vi "QImaging_Main.vi"() -> ()   [LabVIEW 2014]
uses:
  QImaging_Basic/Controls/Readout Speed.ctl
  QImaging_Basic/Controls/Parameter.ctl
  Release/QImaging.dll
panel:
  out "ConfigCam err Readout":i32
  out "ConfigCam err Hi Sens":i32
  in  "High Sensitivity":bool=TRUE
  in  "Readout Speed":T1
  out "Message":string
  in  "Stop Live Preview":bool
  in  "Abort Multi Grab":bool
  in  "Multi Grab":bool
  out "Saturating?":bool
  out "Average":dbl
  out "Std Dev":dbl
  in  "Overwrite?":bool
  in  "Snap current Data":bool
  in  "Save Data":bool
  in  "Racine chemin de sauvegarde":path=path "C:/Users/loa/Documents/DONNEES MANIP GAZ/Hiver 2015"
  out "Warning":bool
  out "Message":string
  in  "Indice":u32
  in  "Nom du fichier":string="tir"
  in  "Mode de Sauvegarde":u16(ring)=1 items=["Manuel", "Automatique"]
  out "Max Val":u16
  out "CCD Height":u32=1 min=1 max=4 step=1
  out "CCD Width":u32=1 min=1 max=4 step=1
  out "Camera Handle":u32
  in  "Abort Frame":bool
  out "sizeOfBuf":u32
  out "errcode":i32
  out "pBuf address":u32
  out "pFrame address":u32
  out "Waiting for Trigger":bool
  in  "Grab Image":bool
  in  "Queue Frame":bool
  in  "Trig":bool
  out "ROI Height":u32=1 min=1 max=4 step=1
  out "ROI Width":u32=1 min=1 max=4 step=1
  in  "Binning":u32=1 min=1 max=4 step=1
  out "ParamVal":u32[](array[numeric])
  out "Open Cam Error":i32
  out "LibCam Error":u32
  out "LibOpen error":i32
  in  "Exposure Time":u32=100
  out "Camera Id":u32
  out "error out":errorcluster
  in  "error in (no error)":errorcluster
  in  "Stop":bool
  out "Captured Image":u16[][](graph)
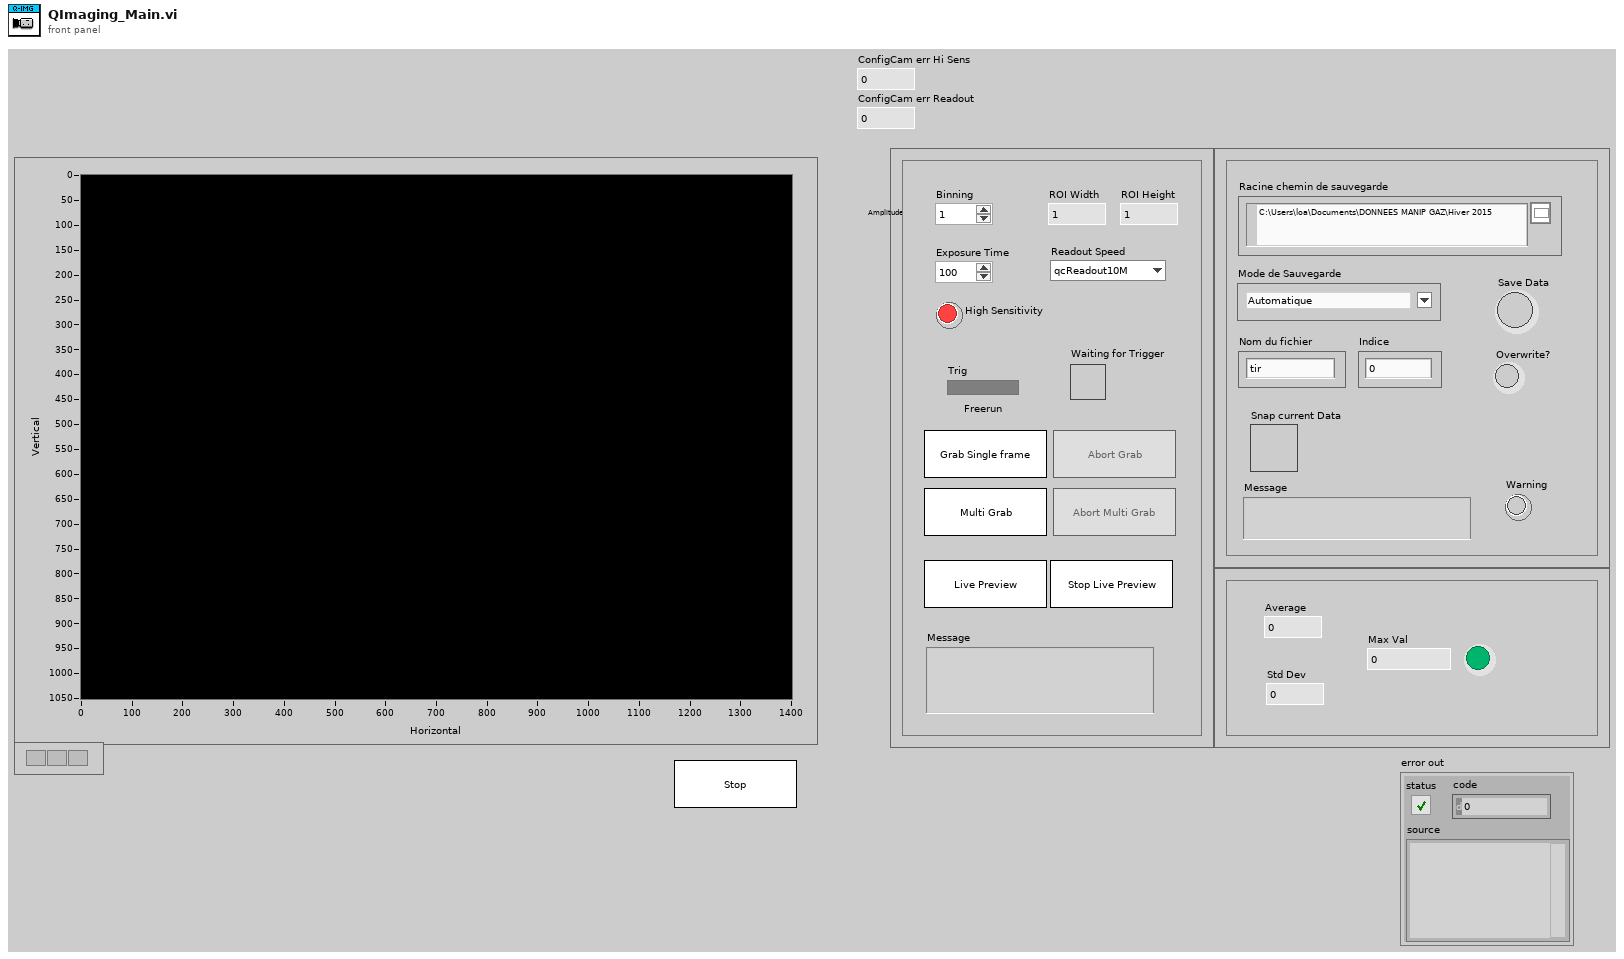
[diagram p1: front panel]
types:
  T1 = typedef "Readout Speed.ctl" = enum16{"qcReadout10M", "qcReadout20M", "qcReadout30M"}
  T2 = enum8{"Enabled", "Disabled", "Disabled and Grayed Out"}
  T3 = typedef "Parameter.ctl" = enum32{"Gain ", "Offset", "Exposure", "Binning", "HzBinning", "VtBinning", "Readout speed", "Trigger Type", "Color Wheel", "Cooler Active", "Exposure red", "Exposure blue", "Image format", "ROI X", "ROI Y", "ROI Width", "ROI Height", "Reserved1", "Shutter State", "Reserved2", "SyncB", "Reserved3", "IntensifierGain (deprecated)", "Trig Delay", "Camera Mode", "Normalized Gain", "Normalized Intensifier Gain", "Do post processing ", "Post Proc Gain Red", "Post Proc Gain Green", "Post Proc Gain Blue", "Post Proc Bayer Algo", "Post Proc Image Format", "Fan Speed", "Blackout Mode", "High Sensitivity Mode", "Readout Port", "EM Gain", "Open Delay Shutter", "Close Delay Shutter", "CCD Clearing Mode", "Over Sample", "Reserved5", "Reserved6", "Reserved7"}
  T4 = typedef "Image Type" = u32
  T5 = typedef "IMAQ Image.ctl" = refnum<image>
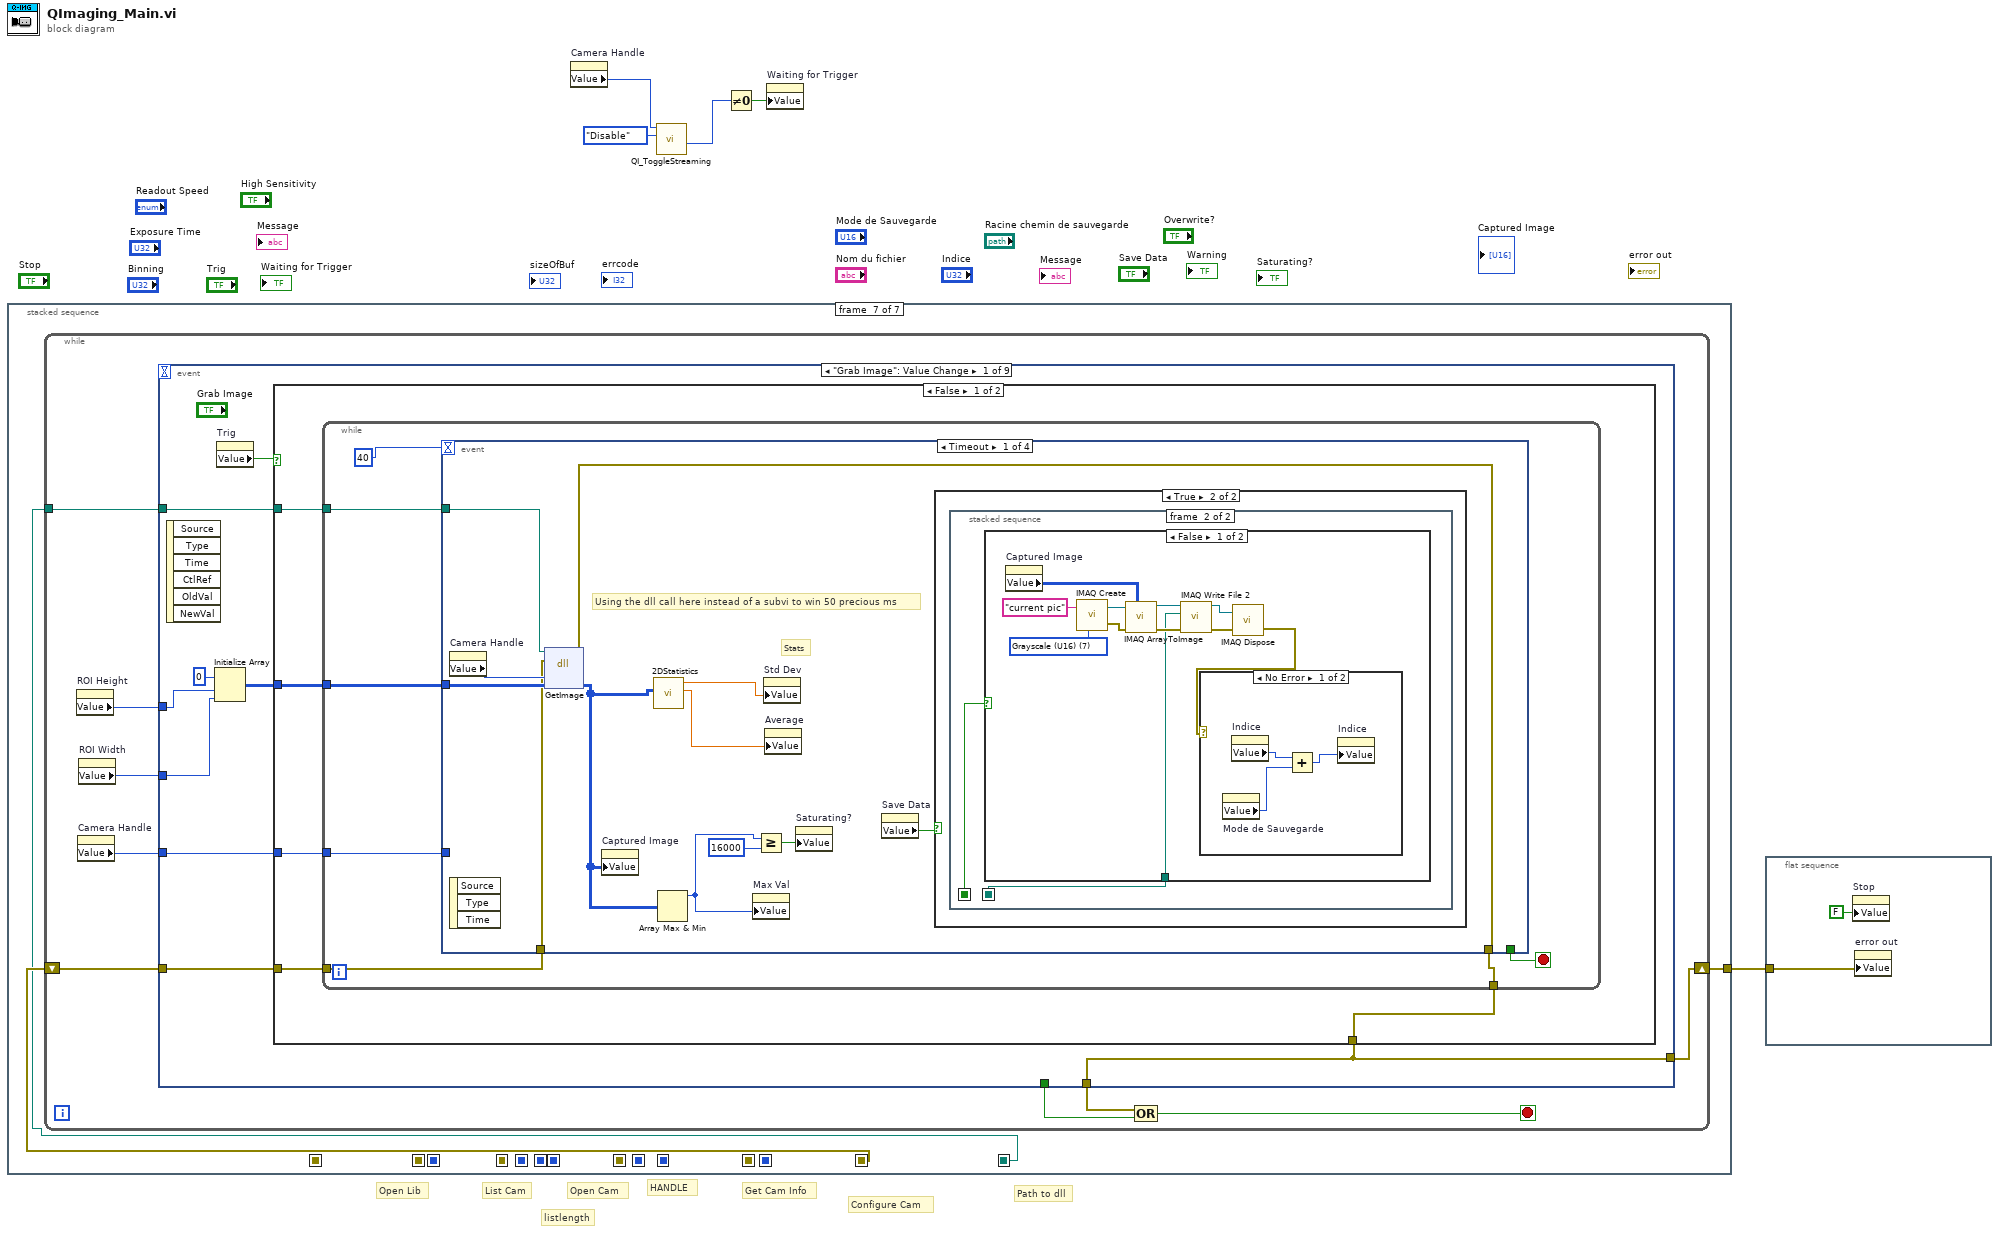
[diagram p0: block diagram]
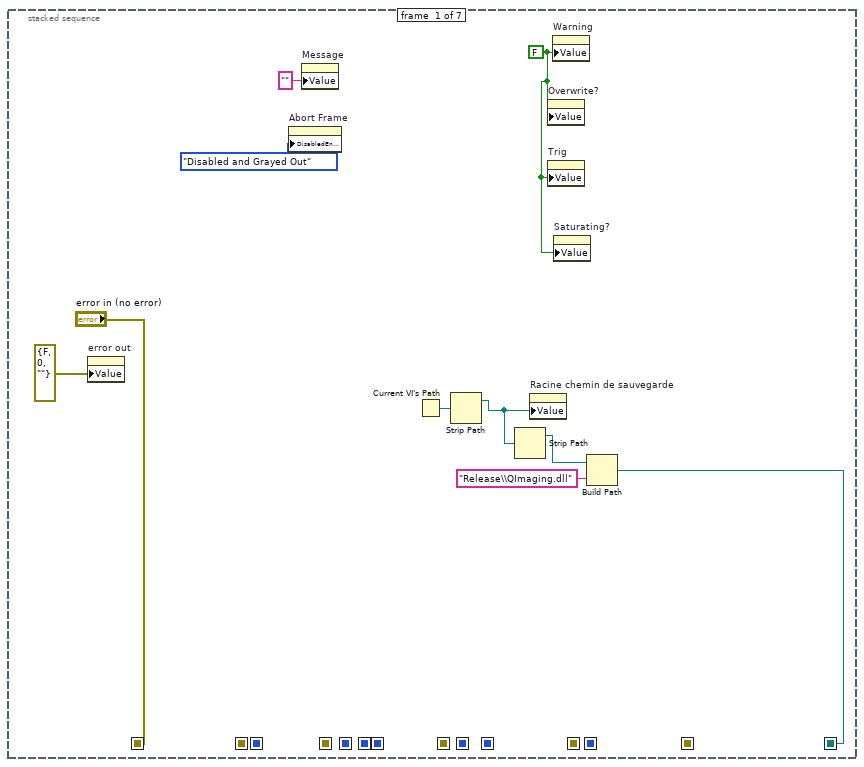
[diagram p2: hidden frame]
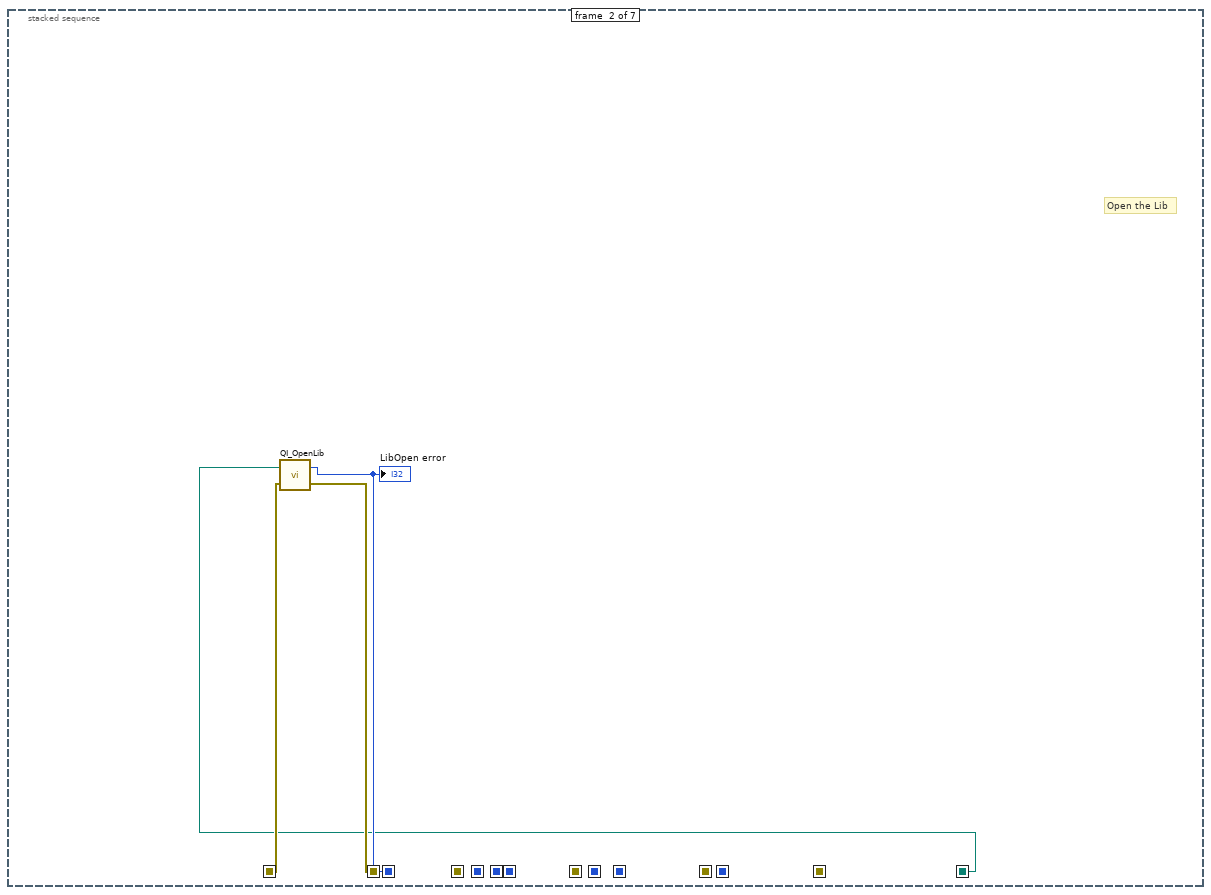
[diagram p3: hidden frame]
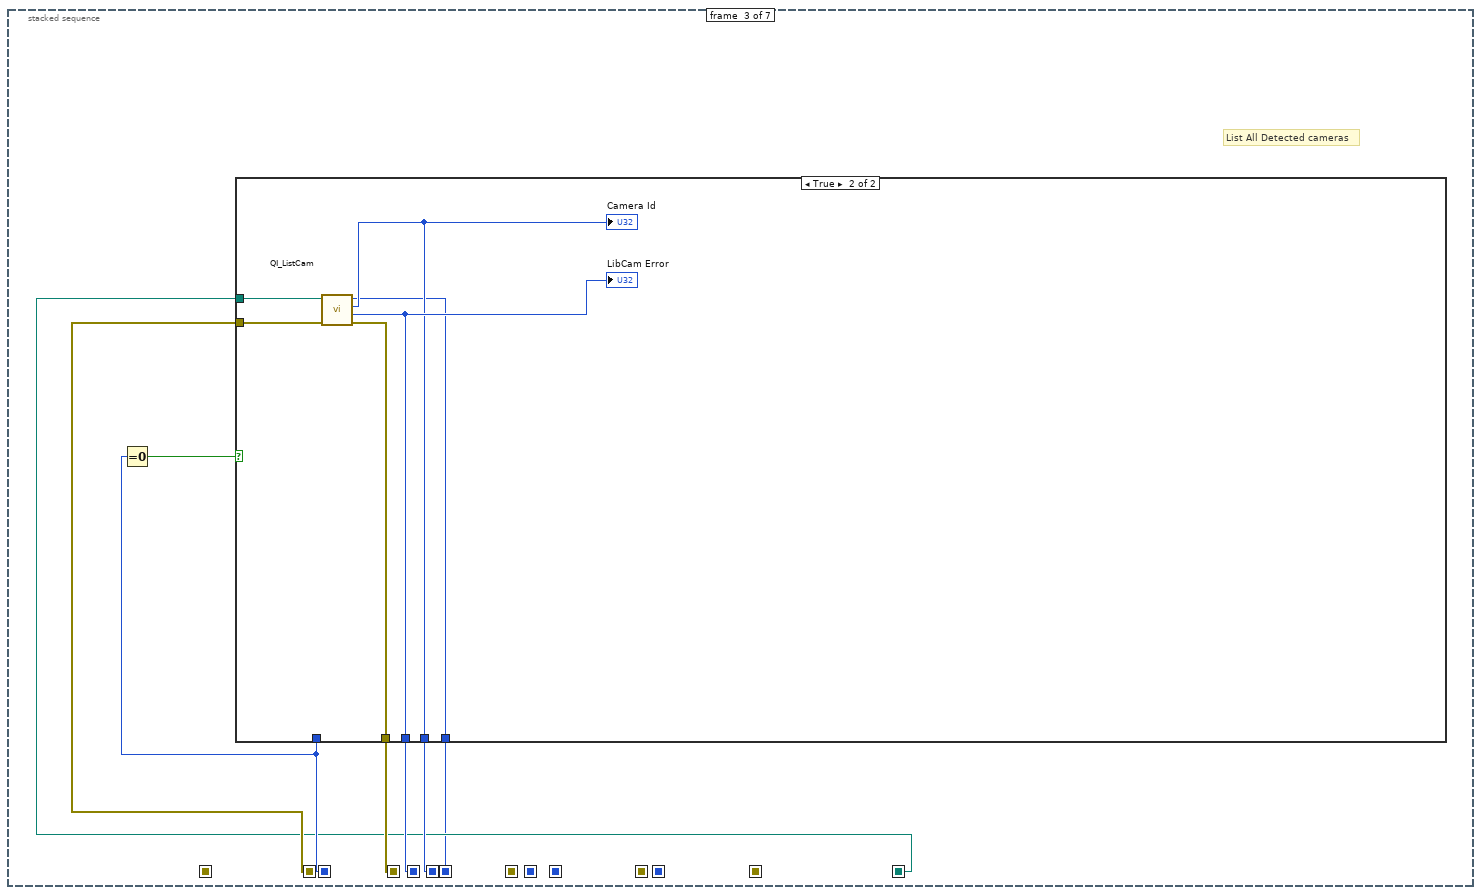
[diagram p4: hidden frame]
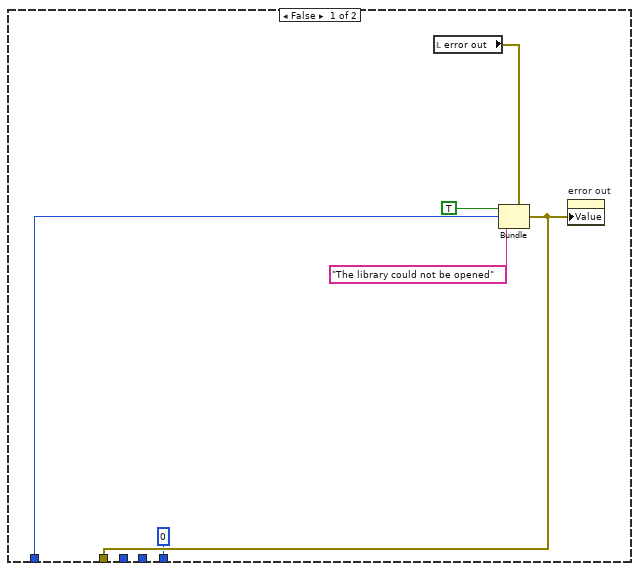
[diagram p5: hidden frame]
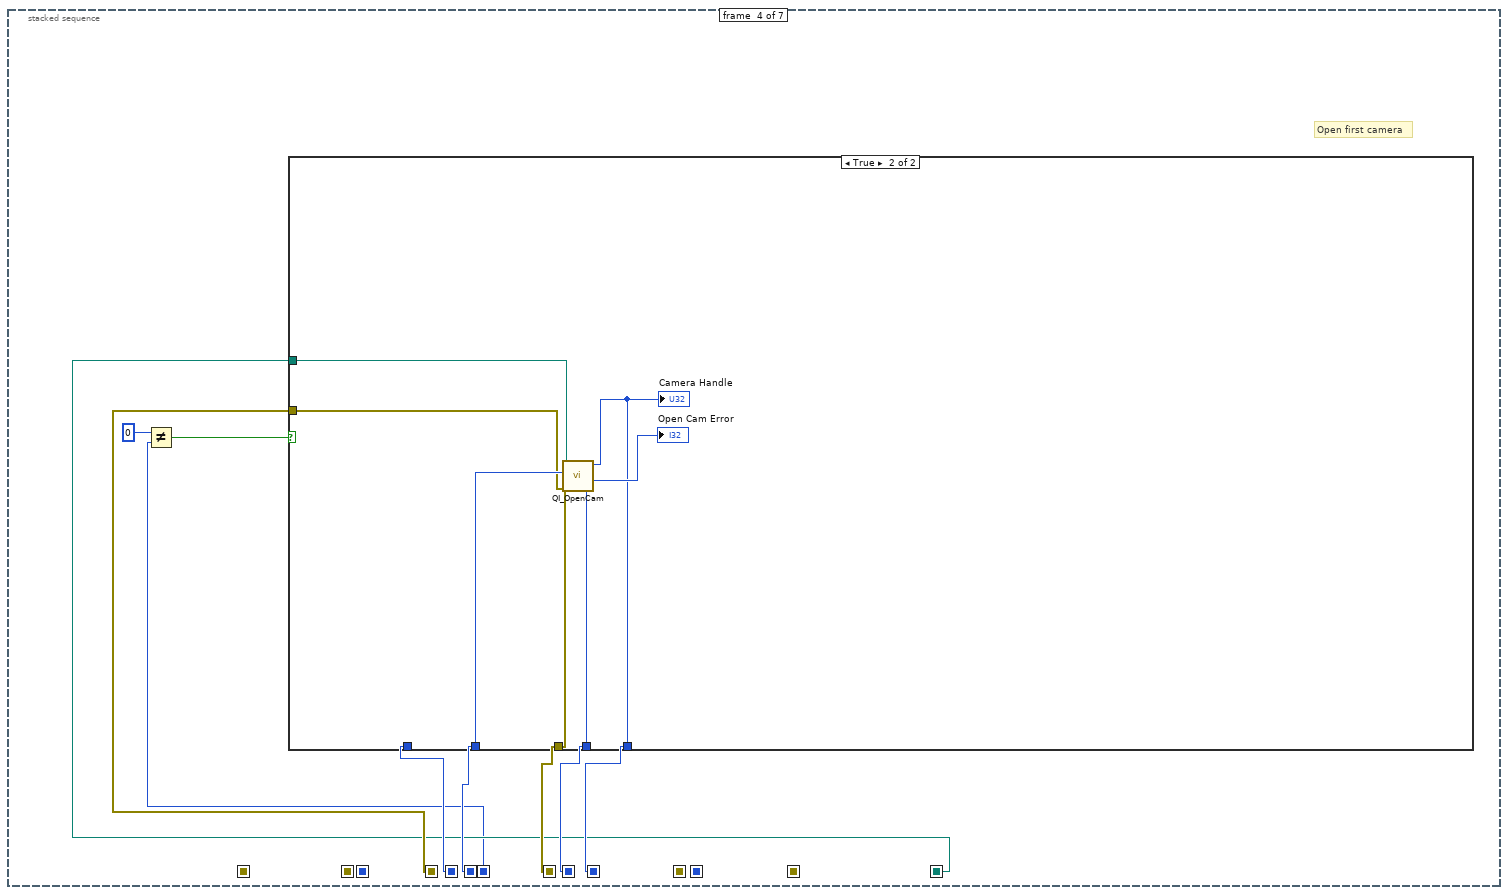
[diagram p6: hidden frame]
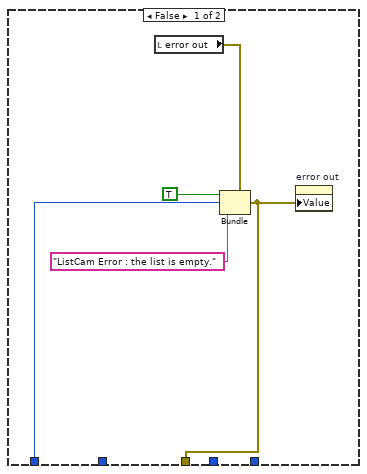
[diagram p7: hidden frame]
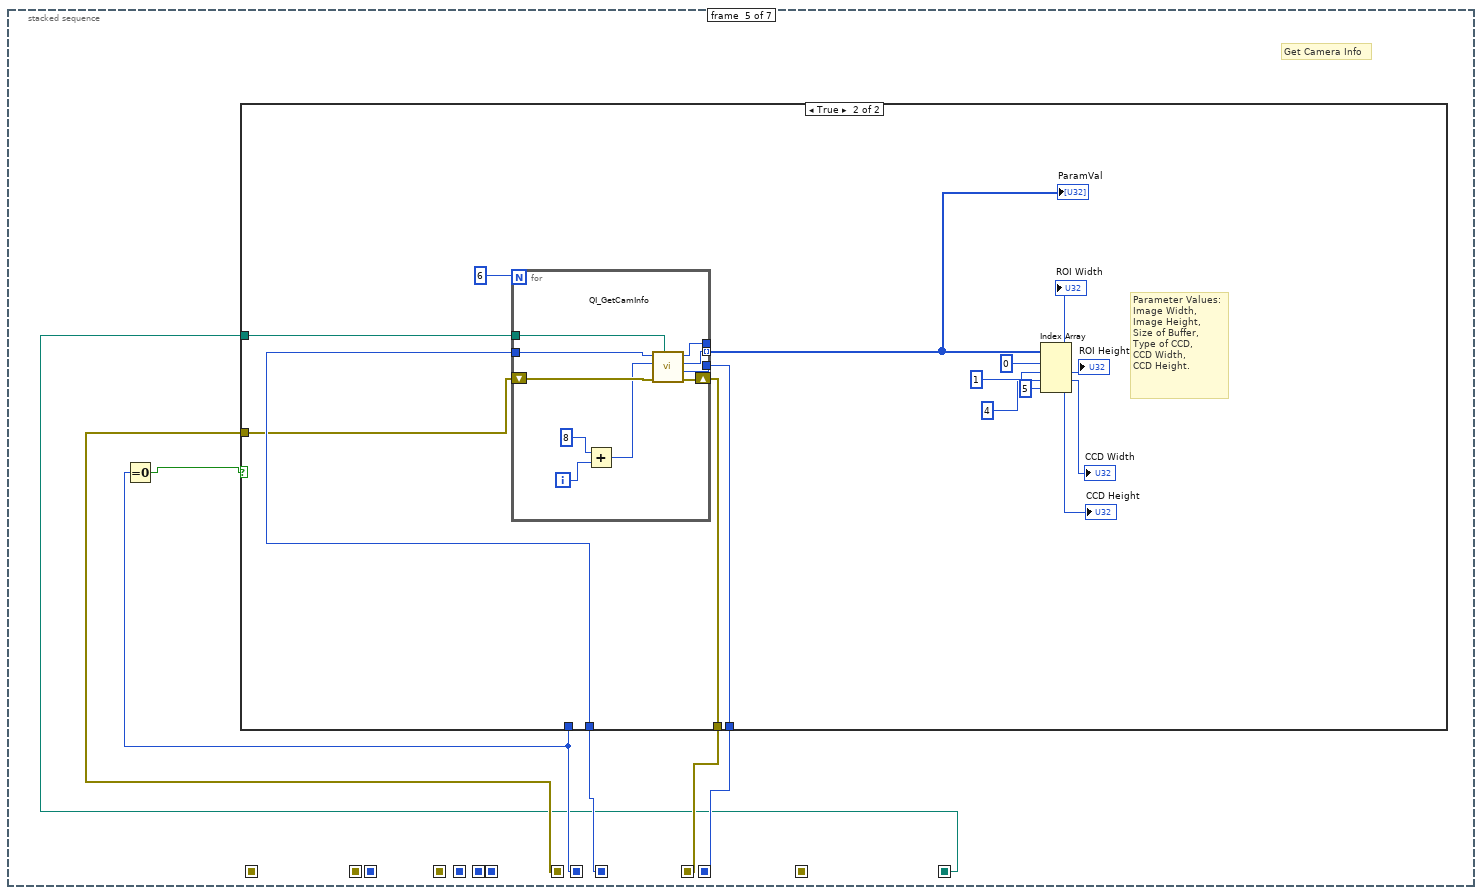
[diagram p8: hidden frame]
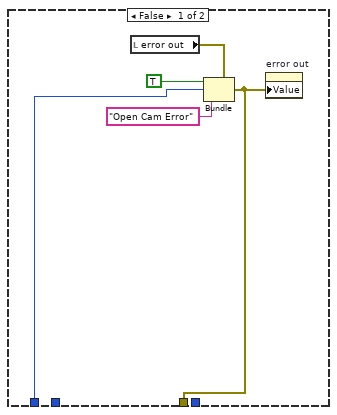
[diagram p9: hidden frame]
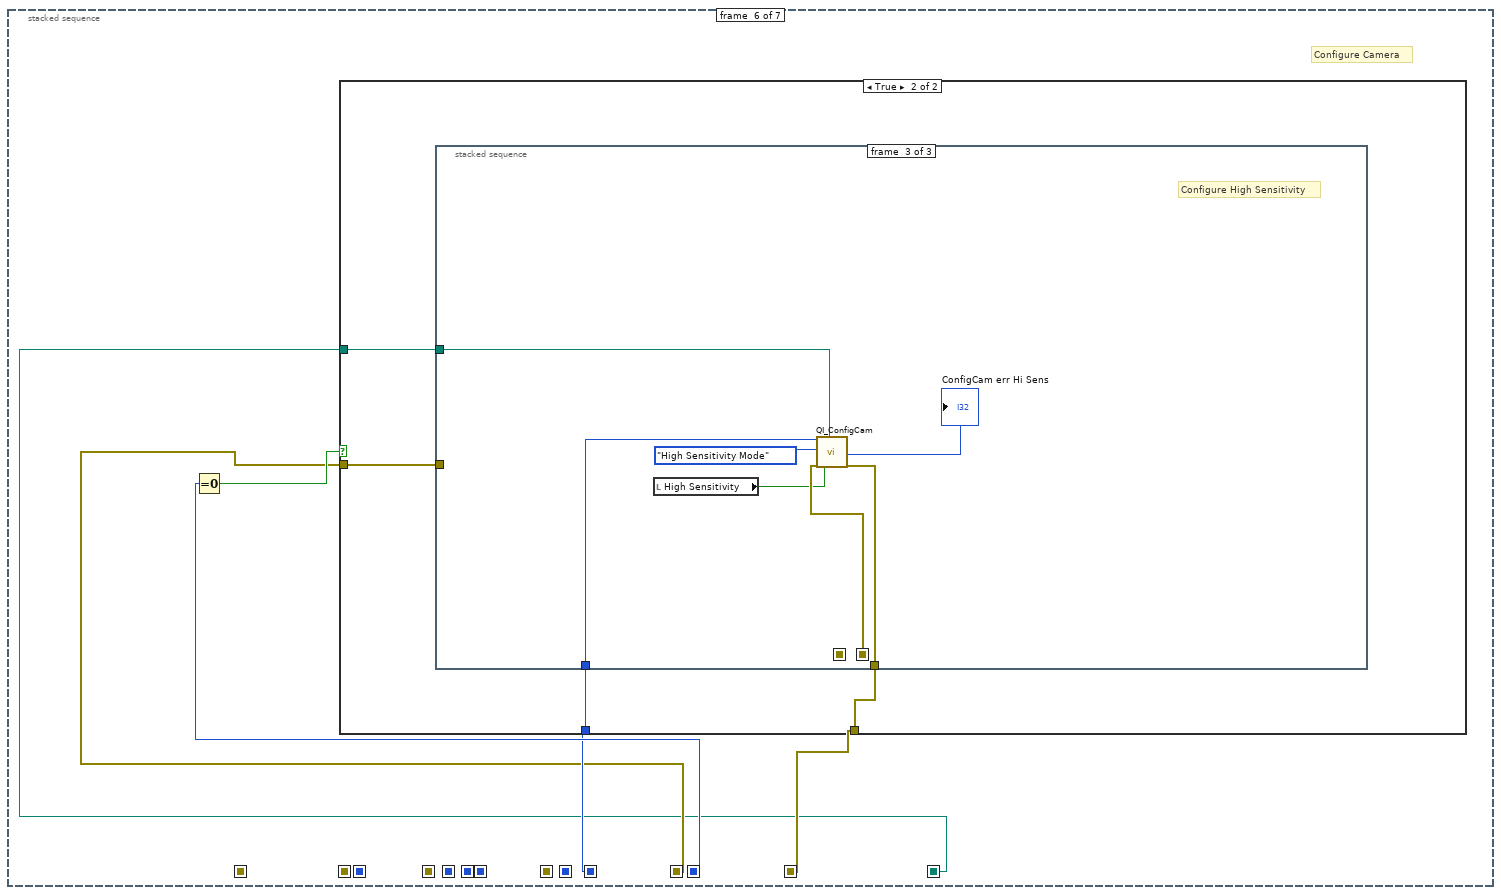
[diagram p10: hidden frame]
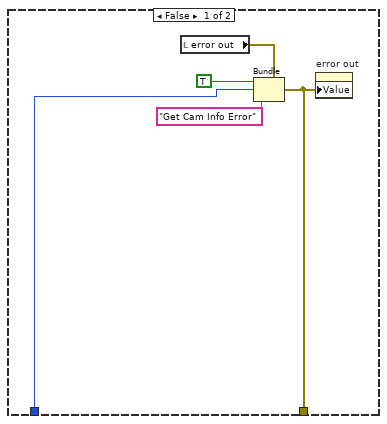
[diagram p11: hidden frame]
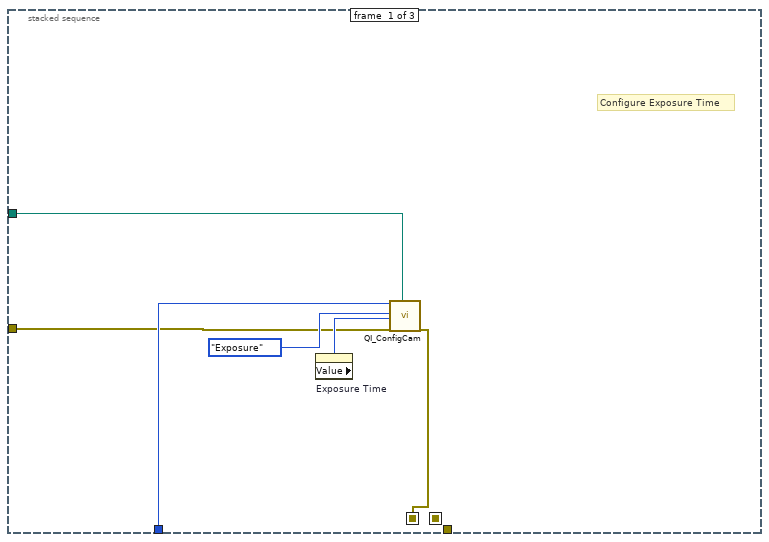
[diagram p12: hidden frame]
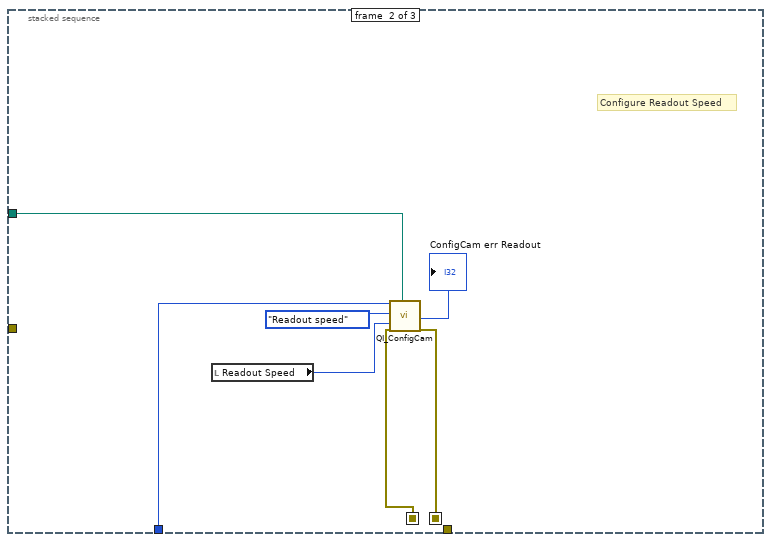
[diagram p13: hidden frame]
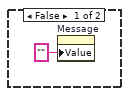
[diagram p14: hidden frame]
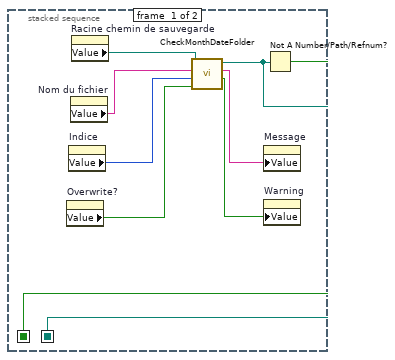
[diagram p15: hidden frame]
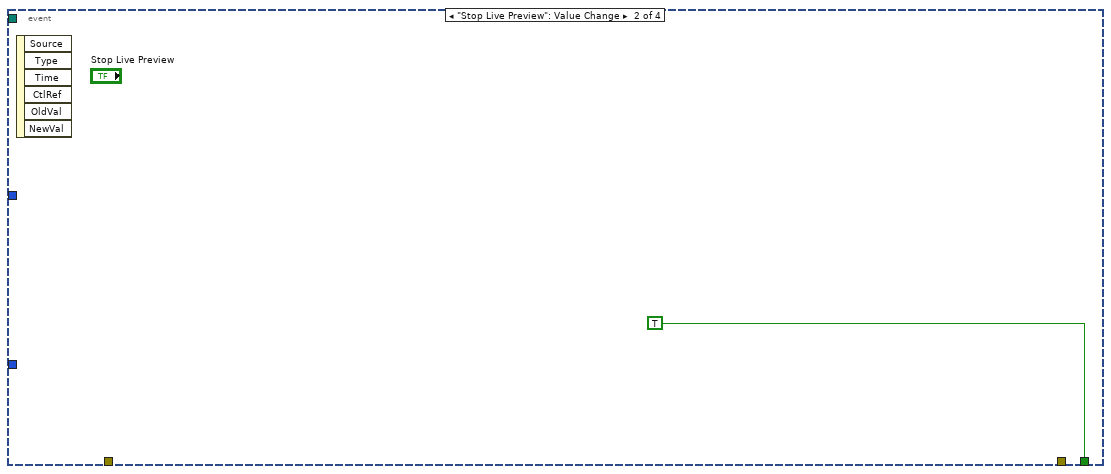
[diagram p18: hidden frame]
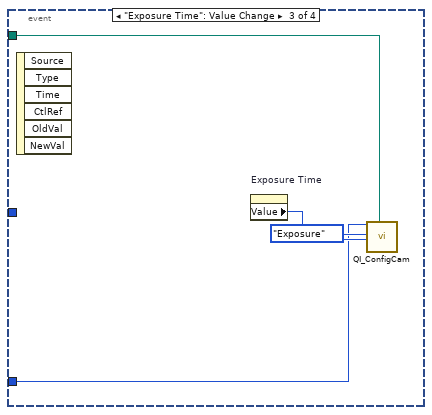
[diagram p19: hidden frame]
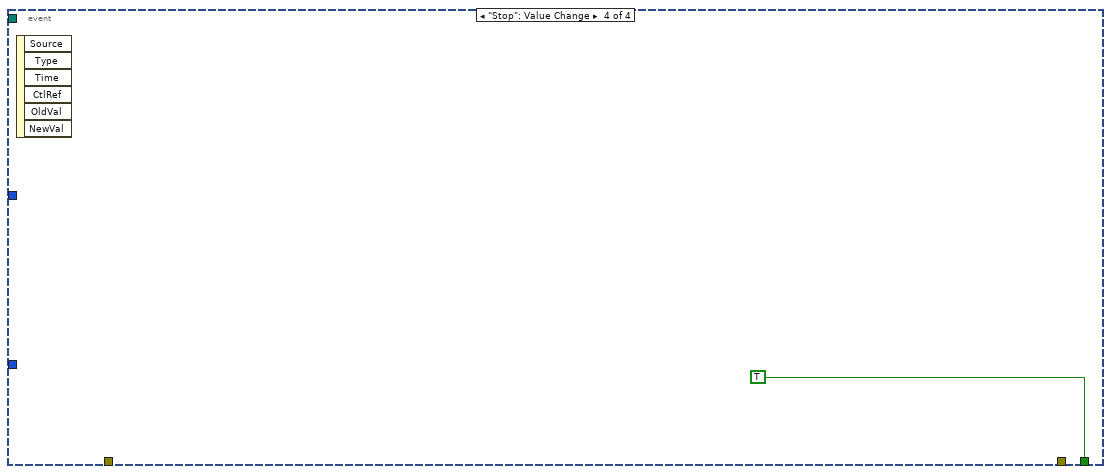
[diagram p20: hidden frame]
diagram:
  # "listlength"
  # "Path to dll"
  # "HANDLE"
  # "Configure Cam"
  # "Get Cam Info"
  # "Open Cam"
  # "List Cam"
  # "Open Lib"
  n1 = stacked-sequence {
    seq-local: [_ w19 _ _ _ _ _] -> [_ _ w22 _ _ _ _]
    seq-local: [_ w18 _ _ _ _ _] -> [_ _ w24 _ _ _ _]
    seq-local: [_ _ w27 _ _ _ _] -> [_ _ _ w43 _ _ _]
    seq-local: [_ _ w26 _ _ _ _] -> [_ _ _ w45 _ _ _]
    seq-local: [_ _ w25 _ _ _ _] -> [_ _ _ w49 _ _ _]
    seq-local: [_ _ _ w48 _ _ _] -> [_ _ _ _ w62 _ _]
    seq-local: [_ _ _ w47 _ _ _] -> [_ _ _ _ w64 _ _]
    seq-local: [_ _ _ w46 _ _ _] -> [_ _ _ _ w67 w102 _]
    seq-local: [_ _ _ _ w66 _ _] -> [_ _ _ _ _ w99 _]
    seq-local: [_ _ _ _ w65 _ _] -> [_ _ _ _ _ w103 _]
    seq-local: [_ _ _ _ _ w101 _] -> [_ _ _ _ _ _ w135]
    seq-local: ["error in (no error)" _ _ _ _ _ _] -> [_ w17 _ _ _ _ _]
    seq-local: [w6 _ _ _ _ _ _] -> [_ w16 w21 w42 w61 w98 w133]
    seq-local: [_ _ w20 _ _ _ _] -> [_ _ _ w41 _ _ _]
    tunnel: [_ _ _ _ _ _ w134] -> w5
    frame #0 {
      w11 = FALSE ("Warning")
      n2 = property on="error out" class="Clust (strict)"("Value"=errorcluster {"status"=FALSE, "code"=0, "source"=""} ("error in (no error)")) -> ()  [unwired: 2 in, 2 out]
      n3 = property on="Abort Frame" class="Bool"("DisabledEnum"=T2."Disabled and Grayed Out" ("Disabled")) -> ()  [unwired: 2 in, 2 out]
      n4 = property on="Message" class="Str"("Value"="" ("Message")) -> ()  [unwired: 2 in, 2 out]
      n5 = Current VI's Path() -> (path=w10:path)
      n6 = Strip Path(path=w10) -> (stripped path=w9:path)  [unwired: 1 out]
      n7 = Strip Path(path=w9) -> (stripped path=w8:path)  [unwired: 1 out]
      n8 = property on="Racine chemin de sauvegarde" class="Path"("Value"=w9) -> ()  [unwired: 2 in, 2 out]
      n9 = property on="Overwrite?" class="Bool (strict)"("Value"=w11) -> ()  [unwired: 2 in, 2 out]
      n10 = property on="Trig" class="Bool (strict)"("Value"=w11) -> ()  [unwired: 2 in, 2 out]
      n11 = property on="Warning" class="Bool (strict)"("Value"=w11) -> ()  [unwired: 2 in, 2 out]
      n12 = property on="Saturating?" class="Bool (strict)"("Value"=w11) -> ()  [unwired: 2 in, 2 out]
      n13 = Build Path(base path=w8, name or relative path="Release\\QImaging.dll") -> (appended path=w6:path)
    }
    frame #1 {
      # "Open the Lib"
      n14 = call "QI_OpenLib.vi"("error in (no error)"=w17, "path to dll"=w16) -> ("error out"=w19:errorcluster, "LibOpen error"=w18:i32)
      "LibOpen error" <- w18
    }
    frame #2 {
      # "List All Detected cameras"
      n15 = Equal To 0?(x=w24) -> (x = 0?=w23:bool)
      n16 = case shown="True" w23 {
        tunnel: w24 -> [w30 _]
        tunnel: [w29 w39] -> w27
        tunnel: [_ w38] -> w26
        tunnel: [_ w37] -> w25
        tunnel: w22 -> [_ w36]
        tunnel: w21 -> [_ w35]
        tunnel: [u32 0 ("listLength") w34] -> w20
        frame False {
          n17 = local read "error out"() -> (w31:errorcluster)
          n18 = Bundle(cluster=w31, "status"=TRUE, "code"=w30, "source"="The library could not be opened") -> (w29:errorcluster)
          n19 = property on="error out" class="Clust (strict)"("Value"=w29) -> ()  [unwired: 2 in, 2 out]
        }
        frame True {
          n20 = call "QI_ListCam.vi"("error in (no error)"=w36, "path to dll"=w35) -> ("error out"=w39:errorcluster, "LibCam Error"=w38:u32, "cameraId"=w37:u32, "listLength"=w34:u32)  [unwired: 6 in]
          "Camera Id" <- w37
          "LibCam Error" <- w38
        }
      }
    }
    frame #3 {
      # "Open first camera"
      n21 = Not Equal?(x=u32 0, y=w41) -> (x != y?=w44:bool)
      n22 = case shown="True" w44 {
        tunnel: w49 -> [_ w60]
        tunnel: [w50 w59] -> w48
        tunnel: [_ w58] -> w47
        tunnel: [_ w57] -> w46
        tunnel: w45 -> [w51 _]
        tunnel: w43 -> [_ w56]
        tunnel: w42 -> [_ w55]
        frame False {
          n23 = local read "error out"() -> (w52:errorcluster)
          n24 = Bundle(cluster=w52, "status"=TRUE, "code"=w51, "source"="ListCam Error : the list is empty.") -> (w50:errorcluster)
          n25 = property on="error out" class="Clust (strict)"("Value"=w50) -> ()  [unwired: 2 in, 2 out]
        }
        frame True {
          n26 = call "QI_OpenCam.vi"("error in (no error)"=w56, "Camera ID"=w60, "path to dll"=w55) -> ("error out"=w59:errorcluster, "Open Cam Error"=w58:i32, "Camera Handle"=w57:u32)  [unwired: 6 in]
          "Camera Handle" <- w57
          "Open Cam Error" <- w58
        }
      }
    }
    frame #4 {
      # "Get Camera Info"
      n27 = Equal To 0?(x=w64) -> (x = 0?=w63:bool)
      n28 = case shown="True" w63 {
        tunnel: w67 -> [_ w82]
        tunnel: [w68 w81] -> w66
        tunnel: w64 -> [w69 _]
        tunnel: [_ w80] -> w65
        tunnel: w62 -> [_ w79]
        tunnel: w61 -> [_ w73]
        frame False {
          n29 = local read "error out"() -> (w70:errorcluster)
          n30 = Bundle(cluster=w70, "status"=TRUE, "code"=w69, "source"="Open Cam Error") -> (w68:errorcluster)
          n31 = property on="error out" class="Clust (strict)"("Value"=w68) -> ()  [unwired: 2 in, 2 out]
        }
        frame True {
          # "Parameter Values:\nImage Width,\nImage Height,\nSize of Buffer,\nType of CCD,\nCCD Width,\nCCD Height."
          n32 = for {
            N: 6 -> [_]
            shift-right: [w93] -> w81
            shift-left: w79 -> [w97]
            tunnel: [w92] -> _
            tunnel: [w91] -> w84 mode=indexing
            tunnel: [w90] -> w80
            tunnel: w82 -> [w89]
            tunnel: w73 -> [w88]
            i -> [w96]
            n33 = Add(x=u32 8, y=w96) -> (x+y=w94:u32)
            n34 = call "QI_GetCamInfo.vi"("path to dll"=w88, "error in (no error)"=w97, "paramKey"=w94, "Camera Handle"=w89) -> ("error out"=w93:errorcluster, "CamInfo err"=w90:i32, "paramVal"=w91:u32, "Camera Handle"=w92:u32)  [unwired: 4 in]
          }
          "ParamVal" <- w84
          n35 = Index Array(array=w84, index #1=0 ("index"), index #2=1 ("index"), index #3=4 ("index"), index #4=5 ("index")) -> (element #1=→"ROI Width":u32, element #2=→"ROI Height":u32, element #3=→"CCD Width":u32, element #4=→"CCD Height":u32)
        }
      }
    }
    frame #5 {
      # "Configure Camera"
      n36 = Equal To 0?(x=w103) -> (x = 0?=w100:bool)
      n37 = case shown="True" w100 {
        tunnel: w102 -> [w105 w112]
        tunnel: [w104 w109] -> w101
        tunnel: w99 -> [_ w111]
        tunnel: w98 -> [_ w110]
        frame False {
          n38 = local read "error out"() -> (w106:errorcluster)
          n39 = Bundle(cluster=w106, "status"=TRUE, "code"=w105, "source"="Get Cam Info Error") -> (w104:errorcluster)
          n40 = property on="error out" class="Clust (strict)"("Value"=w104) -> ()  [unwired: 2 in, 2 out]
        }
        frame True {
          n41 = stacked-sequence {
            seq-local: [w113 _ _] -> [_ w122 _]
            seq-local: [_ w121 _] -> [_ _ w129]
            tunnel: w112 -> [w116 w124 w131]
            tunnel: w111 -> [w115 _ _]
            tunnel: w110 -> [w114 w123 w130]
            tunnel: [_ _ w128] -> w109
            frame #0 {
              # "Configure Exposure Time"
              n42 = property on="Exposure Time" class="DigNum (strict)"() -> ("Value"=w117:u32)  [unwired: 2 in, 2 out]
              n43 = call "QI_ConfigCam.vi"("Camera Handle"=w116, "Parameter"=Parameter."Exposure", "paramVal"=w117, "error in (no error)"=w115, "path to dll"=w114) -> ("error out"=w113:errorcluster)  [unwired: 12 in, 2 out]
            }
            frame #1 {
              # "Configure Readout Speed"
              n44 = local read "Readout Speed"() -> (w120:T1)
              n45 = call "QI_ConfigCam.vi"("Camera Handle"=w124, "Parameter"=Parameter."Readout speed", "Readout Speed"=w120, "error in (no error)"=w122, "path to dll"=w123) -> ("ConfigCam err"=→"ConfigCam err Readout":i32, "error out"=w121:errorcluster)  [unwired: 12 in, 1 out]
            }
            frame #2 {
              # "Configure High Sensitivity"
              n46 = local read "High Sensitivity"() -> (w127:bool)
              n47 = call "QI_ConfigCam.vi"("Camera Handle"=w131, "Parameter"=Parameter."High Sensitivity Mode", "error in (no error)"=w129, "High Sensitivity"=w127, "path to dll"=w130) -> ("ConfigCam err"=→"ConfigCam err Hi Sens":i32, "error out"=w128:errorcluster)  [unwired: 12 in, 1 out]
            }
          }
        }
      }
    }
    frame #6 {
      n48 = while {
        shift-right: [w143] -> w134
        shift-left: w135 -> [w144]
        tunnel: w133 -> [w136]
        stop <- w139 stop-if-true
        n49 = property on="ROI Height" class="DigNum (strict)"() -> ("Value"=w141:u32)  [unwired: 2 in, 2 out]
        n50 = property on="Camera Handle" class="DigNum (strict)"() -> ("Value"=w142:u32)  [unwired: 2 in, 2 out]
        n51 = property on="ROI Width" class="DigNum (strict)"() -> ("Value"=w140:u32)  [unwired: 2 in, 2 out]
        n52 = event shown="[0] \"Grab Image\": Value Change" {
          selector: _ -> [_ _ _ _ _ _ _ _ _]
          dyn-events: _ -> [_ _ _ _ _ _ _ _ _]
          timeout: _ -> [_ _ _ _ _ _ _ _ _]
          tunnel: w144 -> [w153 _ w244 _ _ w476 w482 w501 w518]
          tunnel: [w152 _ w242 w346 _ w475 w481 w500 w515] -> w143
          tunnel: w142 -> [w151 _ w245 w345 w469 w477 w485 w502 w516]
          tunnel: w141 -> [w148 _ _ _ _ _ _ _ _]
          tunnel: w140 -> [w147 _ _ _ _ _ _ _ _]
          tunnel: [w152 _ _ _ w468 w475 _ w500 w515] -> w138
          tunnel: [_ _ _ _ TRUE _ _ _ _] -> w137
          tunnel: w136 -> [w145 _ w236 w344 w466 w474 w480 w486 w514]
          event "Grab Image": Value Change {
            n53 = event-data() -> ()  [unwired: 1 in, 6 out]
            n54 = Initialize Array(u16 0 ("element"), w148, w147) -> (w146:u16[][])
            n55 = property on="Trig" class="Bool (strict)"() -> ("Value"=w150:bool)  [unwired: 2 in, 2 out]
            n56 = case shown="False" w150 {
              tunnel: w153 -> [w158 w209]
              tunnel: [w155 w209] -> w152
              tunnel: w151 -> [w157 _]
              tunnel: w146 -> [w156 _]
              tunnel: w145 -> [w154 _]
              frame False {
                n57 = while {
                  tunnel: w158 -> [w165]
                  tunnel: w157 -> [w164]
                  tunnel: w156 -> [w161]
                  tunnel: [w160] -> w155
                  tunnel: w154 -> [w159]
                  stop <- w162 stop-if-true
                  n58 = event shown="[0] Timeout" {
                    selector: _ -> [_ _ _ _]
                    dyn-events: _ -> [_ _ _ _]
                    timeout: 40 -> [_ _ _ _]
                    tunnel: w165 -> [w172 _ _ _]
                    tunnel: w164 -> [_ _ w205 _]
                    tunnel: [_ TRUE _ TRUE] -> w162
                    tunnel: w161 -> [w173 _ _ _]
                    tunnel: [w170 _ _ _] -> w160
                    tunnel: w159 -> [w171 _ w204 _]
                    event Timeout {
                      # "Using the dll call here instead of a subvi to win 50 precious ms"
                      # "Stats"
                      n59 = property on="Camera Handle" class="DigNum (strict)"() -> ("Value"=w174:u32)  [unwired: 2 in, 2 out]
                      n60 = event-data() -> ()  [unwired: 1 in, 3 out]
                      n61 = dll-call lib="C:/Users/appli/Documents/Aline/octo-labview/QImaging/Release/QImaging.dll" fn="GetImage"(path in=w171, error in=w172, "handle"=w174, "data"=w173) -> (error out=w170:errorcluster, "data"=w168:u16[][])  [unwired: 3 in, 1 out]
                      n62 = property on="Captured Image" class="IntGraph (strict)"("Value"=w168) -> ()  [unwired: 2 in, 2 out]
                      n63 = call "2DStatistics.vi"("data"=w168) -> ("Average"=w166:dbl, "StDev"=w167:dbl)  [unwired: 9 in]
                      n64 = Array Max & Min(array=w168) -> (max value=w175:u16)  [unwired: 3 out]
                      n65 = property on="Max Val" class="DigNum (strict)"("Value"=w175) -> ()  [unwired: 2 in, 2 out]
                      n66 = Greater Or Equal?(x=w175, y=u16 16000) -> (x >= y?=w176:bool)
                      n67 = property on="Std Dev" class="DigNum (strict)"("Value"=w167) -> ()  [unwired: 2 in, 2 out]
                      n68 = property on="Average" class="DigNum (strict)"("Value"=w166) -> ()  [unwired: 2 in, 2 out]
                      n69 = property on="Saturating?" class="Bool (strict)"("Value"=w176) -> ()  [unwired: 2 in, 2 out]
                      n70 = property on="Save Data" class="Bool (strict)"() -> ("Value"=w169:bool)  [unwired: 2 in, 2 out]
                      n71 = case shown="True" w169 {
                        frame False {
                          n72 = property on="Message" class="Str"("Value"="" ("Message Acquisition")) -> ()  [unwired: 2 in, 2 out]
                        }
                        frame True {
                          n73 = stacked-sequence {
                            seq-local: [w180 _] -> [_ w188]
                            seq-local: [w179 _] -> [_ w187]
                            frame #0 {
                              n74 = property on="Overwrite?" class="Bool (strict)"() -> ("Value"=w181:bool)  [unwired: 2 in, 2 out]
                              n75 = property on="Indice" class="DigNum (strict)"() -> ("Value"=w184:u32)  [unwired: 2 in, 2 out]
                              n76 = property on="Nom du fichier" class="Str"() -> ("Value"=w185:string)  [unwired: 2 in, 2 out]
                              n77 = property on="Racine chemin de sauvegarde" class="Path"() -> ("Value"=w186:path)  [unwired: 2 in, 2 out]
                              n78 = call "CheckMonthDateFolder.vi"("Overwrite?"=w181, "Index"=w184, "File Name"=w185, "Folder Path Control"=w186) -> ("Warning"=w182:bool, "Message"=w183:string, "File Path"=w179:path)  [unwired: 5 in]
                              n79 = property on="Message" class="Str"("Value"=w183) -> ()  [unwired: 2 in, 2 out]
                              n80 = property on="Warning" class="Bool (strict)"("Value"=w182) -> ()  [unwired: 2 in, 2 out]
                              n81 = Not A Number/Path/Refnum?(number/path/refnum=w179) -> (NaN/Path/Refnum?=w180:bool)
                            }
                            frame #1 {
                              n82 = case shown="False" w188 {
                                tunnel: w187 -> [w190 _]
                                frame False {
                                w195 = T4 7 items=["Grayscale (U8)", "Grayscale (I16)", "Grayscale (SGL)", "Complex (CSG)", "RGB (U32)", "HSL (U32)", "RGB (U64)", "Grayscale (U16)"] ("Image Type")
                                n83 = property on="Captured Image" class="IntGraph (strict)"() -> ("Value"=w191:u16[][])  [unwired: 2 in, 2 out]
                                n84 = call "IMAQ Create"("Image Name"="current pic", "Image Type"=w195) -> ("New Image"=w198:T5, "error out"=w192:errorcluster)  [unwired: 3 in]
                                n85 = call "IMAQ ArrayToImage"("Image Pixels (U16)"=w191, "error in (no error)"=w192, "Image"=w198) -> ("error out"=w193:errorcluster, "Image Out"=w199:T5)  [unwired: 7 in]
                                n86 = call-poly "IMAQ Write File 2"("error in (no error)"=w193, "File Path"=w190, "Image"=w199) -> ("error out"=w194:errorcluster, "Image Out (duplicate)"=w197:T5)  [unwired: 7 in]
                                n87 = call "IMAQ Dispose"("Image"=w197, "error in (no error)"=w194) -> ("error out"=w189:errorcluster)  [unwired: 4 in]
                                n88 = case shown="No Error" w189 {
                                frame No Error {
                                n89 = property on="Mode de Sauvegarde" class="Ring (strict)"() -> ("Value"=w201:u16)  [unwired: 2 in, 2 out]
                                n90 = property on="Indice" class="DigNum (strict)"() -> ("Value"=w202:u32)  [unwired: 2 in, 2 out]
                                n91 = Add(x=w202, y=w201) -> (x+y=w200:u32)
                                n92 = property on="Indice" class="DigNum (strict)"("Value"=w200) -> ()  [unwired: 2 in, 2 out]
                                }
                                frame Error {
                                }
                                }
                                }
                                frame True {
                                }
                              }
                            }
                          }
                        }
                      }
                    }
                    event "Stop Live Preview": Value Change {
                      n93 = event-data() -> ()  [unwired: 1 in, 6 out]
                    }
                    event "Exposure Time": Value Change {
                      n94 = event-data() -> ()  [unwired: 1 in, 6 out]
                      n95 = property on="Exposure Time" class="DigNum (strict)"() -> ("Value"=w206:u32)  [unwired: 2 in, 2 out]
                      n96 = call "QI_ConfigCam.vi"("Camera Handle"=w205, "Parameter"=Parameter."Exposure", "paramVal"=w206, "path to dll"=w204) -> ()  [unwired: 13 in, 3 out]
                    }
                    event "Stop": Value Change {
                      n97 = event-data() -> ()  [unwired: 1 in, 6 out]
                    }
                  }
                }
              }
              frame True {
                n98 = property on="Message" class="Str"("Value"="This function is not available when the camera trig is hardware. Use Multi Grab or Grab Single Frame instead. " ("Message Acquisition")) -> ()  [unwired: 2 in, 2 out]
              }
            }
          }
          event "Snap current Data": Value Change {
            n99 = event-data() -> ()  [unwired: 1 in, 6 out]
            n100 = property on="Overwrite?" class="Bool (strict)"() -> ("Value"=w213:bool)  [unwired: 2 in, 2 out]
            n101 = property on="Indice" class="DigNum (strict)"() -> ("Value"=w216:u32)  [unwired: 2 in, 2 out]
            n102 = property on="Nom du fichier" class="Str"() -> ("Value"=w217:string)  [unwired: 2 in, 2 out]
            n103 = property on="Racine chemin de sauvegarde" class="Path"() -> ("Value"=w218:path)  [unwired: 2 in, 2 out]
            n104 = call "CheckMonthDateFolder.vi"("Overwrite?"=w213, "Index"=w216, "File Name"=w217, "Folder Path Control"=w218) -> ("Warning"=w214:bool, "Message"=w215:string, "File Path"=w211:path)  [unwired: 5 in]
            n105 = property on="Message" class="Str"("Value"=w215) -> ()  [unwired: 2 in, 2 out]
            n106 = property on="Warning" class="Bool (strict)"("Value"=w214) -> ()  [unwired: 2 in, 2 out]
            n107 = Not A Number/Path/Refnum?(number/path/refnum=w211) -> (NaN/Path/Refnum?=w212:bool)
            n108 = case shown="False" w212 {
              tunnel: w211 -> [w219 _]
              frame False {
                n109 = stacked-sequence {
                  seq-local: [w222 _] -> [_ w231]
                  tunnel: w219 -> [w221 _]
                  frame #0 {
                    w226 = T4 7 items=["Grayscale (U8)", "Grayscale (I16)", "Grayscale (SGL)", "Complex (CSG)", "RGB (U32)", "HSL (U32)", "RGB (U64)", "Grayscale (U16)"] ("Image Type")
                    n110 = property on="Captured Image" class="IntGraph (strict)"() -> ("Value"=w220:u16[][])  [unwired: 2 in, 2 out]
                    n111 = call "IMAQ Create"("Image Name"="current pic", "Image Type"=w226) -> ("New Image"=w229:T5, "error out"=w223:errorcluster)  [unwired: 3 in]
                    n112 = call "IMAQ ArrayToImage"("Image Pixels (U16)"=w220, "error in (no error)"=w223, "Image"=w229) -> ("error out"=w224:errorcluster, "Image Out"=w230:T5)  [unwired: 7 in]
                    n113 = call-poly "IMAQ Write File 2"("error in (no error)"=w224, "File Path"=w221, "Image"=w230) -> ("error out"=w225:errorcluster, "Image Out (duplicate)"=w228:T5)  [unwired: 7 in]
                    n114 = call "IMAQ Dispose"("Image"=w228, "error in (no error)"=w225) -> ("error out"=w222:errorcluster)  [unwired: 4 in]
                  }
                  frame #1 {
                    n115 = case shown="No Error" w231 {
                      frame No Error {
                        n116 = property on="Mode de Sauvegarde" class="Ring (strict)"() -> ("Value"=w233:u16)  [unwired: 2 in, 2 out]
                        n117 = property on="Indice" class="DigNum (strict)"() -> ("Value"=w234:u32)  [unwired: 2 in, 2 out]
                        n118 = Add(x=w234, y=w233) -> (x+y=w232:u32)
                        n119 = property on="Indice" class="DigNum (strict)"("Value"=w232) -> ()  [unwired: 2 in, 2 out]
                      }
                      frame Error {
                      }
                    }
                  }
                }
              }
              frame True {
              }
            }
          }
          event "Queue Frame": Value Change {
            n120 = event-data() -> ()  [unwired: 1 in, 6 out]
            n121 = call "QI_ToggleStreaming.vi"("path to dll"=w236, "error in (no error)"=w244, "Enable?"=enum16{"Disable", "Enable"}."Enable", "Camera Handle"=w245) -> ("error out"=w247:errorcluster, "enable"=w240:u32, "Camera Handle"=w246:u32)  [unwired: 4 in, 1 out]
            n122 = flat-sequence {
              tunnel: w236 -> [w255]
              tunnel: [w255] -> w235
              frame #0 {
                n123 = property on="Abort Frame" class="Bool"("DisabledEnum"=T2."Enabled" ("Disabled")) -> ()  [unwired: 2 in, 2 out]
              }
            }
            n124 = Not Equal To 0?(x=w240) -> (x != 0?=w241:bool)
            n125 = Create User Event(user event datatype="" ("stringMessage")) -> (user event=w250:refnum<user-event>)  [unwired: 1 in, 1 out]
            n126 = property on="Waiting for Trigger" class="Bool (strict)"("Value"=w241) -> ()  [unwired: 2 in, 2 out]
            n127 = register-events(w250) -> (reference out=w253:refnum<event-registration>)  [unwired: 2 in, 1 out]
            n128 = call "QI_AsyncGrab.vi"("path to dll"=w236, "error in (no error)"=w247, "UserEventRef"=w250, "Camera Handle"=w246) -> ("error out"=w248:errorcluster, "Frame Address"=→"pFrame address":u32, "Buffer Address"=→"pBuf address":u32)  [unwired: 4 in, 1 out]
            n129 = property on="ROI Width" class="DigNum (strict)"() -> ("Value"=w238:u32)  [unwired: 2 in, 2 out]
            n130 = property on="ROI Height" class="DigNum (strict)"() -> ("Value"=w239:u32)  [unwired: 2 in, 2 out]
            n131 = Initialize Array(u16 0 ("element"), w239, w238) -> (w251:u16[][])
            n132 = while {
              tunnel: w253 -> [w263]
              tunnel: w251 -> [w260]
              tunnel: w248 -> [w259]
              tunnel: [w258] -> w242
              tunnel: w235 -> [w257]
              stop <- w261 stop-if-true
              n133 = event shown="[0] <stringMessage>: User Event" {
                selector: w263 -> [_ _]
                dyn-events: [_ _] -> w262
                timeout: _ -> [_ _]
                tunnel: [TRUE TRUE] -> w261
                tunnel: w260 -> [w266 _]
                tunnel: w259 -> [w265 w341]
                tunnel: [w264 w336] -> w258
                tunnel: w257 -> [_ w332]
                event User Event {
                  n134 = event-data() -> ()  [unwired: 1 in, 1 out]
                  n135 = stacked-sequence {
                    seq-local: [_ w269 _ _ _ _] -> [_ _ _ _ w282 w325]
                    tunnel: w266 -> [_ w272 _ _ _ _]
                    tunnel: w265 -> [_ _ _ w279 _ _]
                    tunnel: [_ _ _ w278 _ _] -> w264
                    frame #0 {
                      # "Wait until image is available from driver"
                      n136 = Wait (ms)(milliseconds to wait=u32 200) -> ()  [unwired: 1 out]
                    }
                    frame #1 {
                      # "Get data to interface"
                      n137 = property on="ROI Width" class="DigNum (strict)"() -> ("Value"=w270:u32)  [unwired: 2 in, 2 out]
                      n138 = property on="ROI Height" class="DigNum (strict)"() -> ("Value"=w271:u32)  [unwired: 2 in, 2 out]
                      n139 = property on="pBuf address" class="DigNum (strict)"() -> ("Value"=w273:u32)  [unwired: 2 in, 2 out]
                      n140 = dll-call lib="Z:/Programmes en Developpement/QImaging/Release/QImaging.dll" fn="GetFrame"("width"=w270, "height"=w271, "pBuf"=w273, "data"=w272) -> ("data"=w269:u16[][])  [unwired: 7 in, 2 out]
                      n141 = property on="Captured Image" class="IntGraph (strict)"("Value"=w269) -> ()  [unwired: 2 in, 2 out]
                    }
                    frame #2 {
                      # "ALWAYS free memory\nafter calling Async Grab\n(calls malloc)"
                      n142 = property on="pBuf address" class="DigNum (strict)"() -> ("Value"=w274:u32)  [unwired: 2 in, 2 out]
                      n143 = property on="pFrame address" class="DigNum (strict)"() -> ("Value"=w275:u32)  [unwired: 2 in, 2 out]
                      n144 = dll-call lib="Z:/Programmes en Developpement/QImaging/Release/QImaging.dll" fn="RemFrame"("pFrame"=w275, "pBuf"=w274) -> ()  [unwired: 6 in, 2 out]
                    }
                    frame #3 {
                      # "Disable Streaming"
                      n145 = property on="Camera Handle" class="DigNum (strict)"() -> ("Value"=w280:u32)  [unwired: 2 in, 2 out]
                      n146 = call "QI_ToggleStreaming.vi"("error in (no error)"=w279, "Enable?"=enum16{"Disable", "Enable"}."Disable", "Camera Handle"=w280) -> ("error out"=w278:errorcluster, "enable"=w276:u32)  [unwired: 5 in, 2 out]
                      n147 = Not Equal To 0?(x=w276) -> (x != 0?=w277:bool)
                      n148 = property on="Waiting for Trigger" class="Bool (strict)"("Value"=w277) -> ()  [unwired: 2 in, 2 out]
                    }
                    frame #4 {
                      # "Save data"
                      n149 = property on="Save Data" class="Bool (strict)"() -> ("Value"=w283:bool)  [unwired: 2 in, 2 out]
                      n150 = case shown="True" w283 {
                        tunnel: w282 -> [_ w289]
                        frame False {
                        }
                        frame True {
                          n151 = property on="Indice" class="DigNum (strict)"() -> ("Value"=w292:u32)  [unwired: 2 in, 2 out]
                          n152 = property on="Overwrite?" class="Bool (strict)"() -> ("Value"=w293:bool)  [unwired: 2 in, 2 out]
                          n153 = property on="Nom du fichier" class="Str"() -> ("Value"=w291:string)  [unwired: 2 in, 2 out]
                          n154 = property on="Racine chemin de sauvegarde" class="Path"() -> ("Value"=w290:path)  [unwired: 2 in, 2 out]
                          n155 = call "CheckMonthDateFolder.vi"("Overwrite?"=w293, "Index"=w292, "File Name"=w291, "Folder Path Control"=w290) -> ("Warning"=w295:bool, "Message"=w294:string, "File Path"=w284:path)  [unwired: 5 in]
                          n156 = property on="Message" class="Str"("Value"=w294) -> ()  [unwired: 2 in, 2 out]
                          n157 = property on="Warning" class="Bool (strict)"("Value"=w295) -> ()  [unwired: 2 in, 2 out]
                          n158 = Strip Path(path=w284) -> (stripped path=w285:path)  [unwired: 1 out]
                          n159 = Build Path(base path=w285, name or relative path="Exposure.dat" ("Image Name")) -> (appended path=w286:path)
                          n160 = Not A Number/Path/Refnum?(number/path/refnum=w284) -> (NaN/Path/Refnum?=w288:bool)
                          n161 = case shown="False" w288 {
                            tunnel: w289 -> [w298 _]
                            tunnel: w284 -> [w299 _]
                            tunnel: w286 -> [w297 _]
                            tunnel: w284 -> [w296 _]
                            frame False {
                              n162 = stacked-sequence {
                                seq-local: [w308 _] -> [_ w319]
                                tunnel: w299 -> [w307 _]
                                tunnel: w298 -> [w309 _]
                                tunnel: w297 -> [w306 _]
                                tunnel: w296 -> [_ _]
                                frame #0 {
                                w313 = T4 7 items=["Grayscale (U8)", "Grayscale (I16)", "Grayscale (SGL)", "Complex (CSG)", "RGB (U32)", "HSL (U32)", "RGB (U64)", "Grayscale (U16)"] ("Image Type")
                                n163 = property on="Exposure Time" class="DigNum (strict)"() -> ("Value"=w303:u32)  [unwired: 2 in, 2 out]
                                n164 = property on="Indice" class="DigNum (strict)"() -> ("Value"=w304:u32)  [unwired: 2 in, 2 out]
                                n165 = property on="Nom du fichier" class="Str"() -> ("Value"=w305:string)  [unwired: 2 in, 2 out]
                                n166 = call "SavePictureData.vi"("File Path"=w306, "Exposure"=w303, "Index"=w304, "Name"=w305) -> ("error out"=w302:errorcluster)  [unwired: 7 in]
                                n167 = Unbundle By Name(w302) -> ("status"=w301:bool, "source"=w300:string)
                                n168 = call "IMAQ Create"("Image Name"="", "Image Type"=w313) -> ("New Image"=w316:T5, "error out"=w310:errorcluster)  [unwired: 3 in]
                                n169 = case shown="True" w301 {
                                tunnel: w300 -> [_ w318]
                                frame False {
                                }
                                frame True {
                                n170 = property on="Message" class="Str"("Value"=w318) -> ()  [unwired: 2 in, 2 out]
                                }
                                }
                                n171 = call "IMAQ ArrayToImage"("Image Pixels (U16)"=w309, "error in (no error)"=w310, "Image"=w316) -> ("error out"=w311:errorcluster, "Image Out"=w317:T5)  [unwired: 7 in]
                                n172 = call-poly "IMAQ Write File 2"("error in (no error)"=w311, "File Path"=w307, "Image"=w317) -> ("error out"=w312:errorcluster, "Image Out (duplicate)"=w315:T5)  [unwired: 7 in]
                                n173 = call "IMAQ Dispose"("Image"=w315, "error in (no error)"=w312) -> ("error out"=w308:errorcluster)  [unwired: 4 in]
                                }
                                frame #1 {
                                n174 = case shown="No Error" w319 {
                                frame No Error {
                                # "incrémente si mode \nautomatique et écriture \nok"
                                n175 = property on="Mode de Sauvegarde" class="Ring (strict)"() -> ("Value"=w321:u16)  [unwired: 2 in, 2 out]
                                n176 = property on="Indice" class="DigNum (strict)"() -> ("Value"=w322:u32)  [unwired: 2 in, 2 out]
                                n177 = Add(x=w322, y=w321) -> (x+y=w320:u32)
                                n178 = property on="Indice" class="DigNum (strict)"("Value"=w320) -> ()  [unwired: 2 in, 2 out]
                                }
                                frame Error {
                                }
                                }
                                }
                              }
                            }
                            frame True {
                            }
                          }
                        }
                      }
                    }
                    frame #5 {
                      # "Stats"
                      n179 = call "2DStatistics.vi"("data"=w325) -> ("Average"=→"Average":dbl, "StDev"=→"Std Dev":dbl)  [unwired: 9 in]
                      n180 = Array Max & Min(array=w325) -> (max value=w328:u16)  [unwired: 3 out]
                      "Max Val" <- w328
                      n181 = Greater Or Equal?(x=w328, y=u16 16000) -> (x >= y?=w326:bool)
                      n182 = property on="Saturating?" class="Bool (strict)"("Value"=w326) -> ()  [unwired: 2 in, 2 out]
                      n183 = property on="Abort Frame" class="Bool"("DisabledEnum"=T2."Disabled and Grayed Out" ("Disabled")) -> ()  [unwired: 2 in, 2 out]
                    }
                  }
                }
                event "Abort Frame": Value Change {
                  n184 = event-data() -> ()  [unwired: 1 in, 6 out]
                  n185 = property on="Camera Handle" class="DigNum (strict)"() -> ("Value"=w342:u32)  [unwired: 2 in, 2 out]
                  n186 = call "QI_AbortFrame.vi"("path to dll"=w332, "error in (no error)"=w341, "Camera Handle"=w342) -> ("error out"=w331:errorcluster, "Camera Handle"=w337:u32)  [unwired: 7 in]
                  n187 = property on="pBuf address" class="DigNum (strict)"() -> ("Value"=w333:u32)  [unwired: 2 in, 2 out]
                  n188 = property on="pFrame address" class="DigNum (strict)"() -> ("Value"=w334:u32)  [unwired: 2 in, 2 out]
                  n189 = dll-call lib="C:/Users/loa/Documents/Programmes LV/Cameras/QImaging/Release/QImaging.dll" fn="RemFrame"(path in=w332, error in=w331, "pFrame"=w334, "pBuf"=w333) -> (error out=w330:errorcluster)  [unwired: 4 in, 1 out]
                  n190 = call "QI_ToggleStreaming.vi"("path to dll"=w332, "error in (no error)"=w330, "Enable?"=enum16{"Disable", "Enable"}."Disable", "Camera Handle"=w337) -> ("error out"=w336:errorcluster, "enable"=w338:u32)  [unwired: 4 in, 2 out]
                  n191 = property on="Abort Frame" class="Bool"("DisabledEnum"=T2."Disabled and Grayed Out" ("Disabled")) -> ()  [unwired: 2 in, 2 out]
                  n192 = Not Equal To 0?(x=w338) -> (x != 0?=w339:bool)
                  n193 = property on="Waiting for Trigger" class="Bool (strict)"("Value"=w339) -> ()  [unwired: 2 in, 2 out]
                }
              }
              n194 = Unregister For Events(event registration refnum=w262) -> ()  [unwired: 1 in, 1 out]
            }
          }
          event "Multi Grab": Value Change {
            n195 = event-data() -> ()  [unwired: 1 in, 6 out]
            n196 = stacked-sequence {
              seq-local: [_ w355 _ _] -> [_ _ w364 _]
              seq-local: [_ w354 _ _] -> [_ _ w363 _]
              seq-local: [_ w353 _ _] -> [_ _ w366 _]
              seq-local: [w347 _ _ _] -> [_ _ w362 _]
              tunnel: [_ _ w367 _] -> w346
              tunnel: w345 -> [_ _ w365 _]
              tunnel: w344 -> [_ _ w360 _]
              frame #0 {
                # "Enable Streaming"
                n197 = property on="Camera Handle" class="DigNum (strict)"() -> ("Value"=w348:u32)  [unwired: 2 in, 2 out]
                n198 = call "QI_ToggleStreaming.vi"("Enable?"=enum16{"Disable", "Enable"}."Enable", "Camera Handle"=w348) -> ("error out"=w347:errorcluster, "enable"=w351:u32)  [unwired: 6 in, 2 out]
                n199 = Not Equal To 0?(x=w351) -> (x != 0?=w350:bool)
                n200 = property on="Waiting for Trigger" class="Bool (strict)"("Value"=w350) -> ()  [unwired: 2 in, 2 out]
              }
              frame #1 {
                # "Register for events (callback) and allocate memory"
                n201 = Create User Event(user event datatype="" ("stringMessage")) -> (user event=w353:refnum<user-event>)  [unwired: 1 in, 1 out]
                n202 = register-events(w353) -> (reference out=w354:refnum<event-registration>)  [unwired: 2 in, 1 out]
                n203 = property on="ROI Width" class="DigNum (strict)"() -> ("Value"=w356:u32)  [unwired: 2 in, 2 out]
                n204 = property on="ROI Height" class="DigNum (strict)"() -> ("Value"=w357:u32)  [unwired: 2 in, 2 out]
                n205 = property on="Abort Multi Grab" class="Bool"("DisabledEnum"=T2."Enabled" ("Disabled")) -> ()  [unwired: 2 in, 2 out]
                n206 = Initialize Array(u16 0 ("element"), w357, w356) -> (w355:u16[][])
              }
              frame #2 {
                n207 = while {
                  tunnel: [w378] -> w367
                  tunnel: w366 -> [w375]
                  tunnel: w365 -> [w374]
                  tunnel: w364 -> [w373]
                  tunnel: w363 -> [w372]
                  tunnel: w362 -> [w371]
                  tunnel: [w370] -> w361
                  tunnel: w360 -> [w368]
                  stop <- w369 stop-if-true
                  # "Allocates Memory\nfor frames"
                  n208 = call "QI_AsyncGrab.vi"("path to dll"=w368, "error in (no error)"=w371, "UserEventRef"=w375, "Camera Handle"=w374) -> ("error out"=w379:errorcluster, "Frame Address"=w376:u32, "Buffer Address"=w377:u32)  [unwired: 4 in, 1 out]
                  n209 = property on="pFrame address" class="DigNum (strict)"("Value"=w376) -> ()  [unwired: 2 in, 2 out]
                  n210 = property on="pBuf address" class="DigNum (strict)"("Value"=w377) -> ()  [unwired: 2 in, 2 out]
                  n211 = while {
                    tunnel: w373 -> [w387]
                    tunnel: w379 -> [w386]
                    tunnel: [w385] -> w378
                    tunnel: w372 -> [w384]
                    tunnel: [w383] -> w370
                    tunnel: [w381] -> w369
                    tunnel: w368 -> [w380]
                    stop <- w382 stop-if-true
                    n212 = event shown="[0] <stringMessage>: User Event" {
                      selector: w384 -> [_ _]
                      dyn-events: [_ _] -> w383
                      timeout: _ -> [_ _]
                      tunnel: [TRUE w458] -> w382
                      tunnel: w387 -> [w391 _]
                      tunnel: w386 -> [w390 w455]
                      tunnel: [_ w459] -> w385
                      tunnel: [FALSE w458] -> w381
                      tunnel: w380 -> [w388 w452]
                      event User Event {
                        n213 = event-data() -> ()  [unwired: 1 in, 1 out]
                        n214 = stacked-sequence {
                          seq-local: [_ w395 _ _ _] -> [_ _ _ w403 w448]
                          tunnel: w391 -> [_ w399 _ _ _]
                          tunnel: w390 -> [_ _ _ _ _]
                          tunnel: w388 -> [_ w394 w400 _ _]
                          frame #0 {
                            # "Wait until image is available from driver"
                            n215 = Wait (ms)(milliseconds to wait=u32 200) -> ()  [unwired: 1 out]
                          }
                          frame #1 {
                            # "Get data to interface"
                            n216 = property on="pBuf address" class="DigNum (strict)"() -> ("Value"=w396:u32)  [unwired: 2 in, 2 out]
                            n217 = property on="ROI Width" class="DigNum (strict)"() -> ("Value"=w397:u32)  [unwired: 2 in, 2 out]
                            n218 = property on="ROI Height" class="DigNum (strict)"() -> ("Value"=w398:u32)  [unwired: 2 in, 2 out]
                            n219 = dll-call lib="C:/Users/appli/Documents/Aline/octo-labview/QImaging/Release/QImaging.dll" fn="GetFrame"(path in=w394, "width"=w397, "height"=w398, "pBuf"=w396, "data"=w399) -> ("data"=w395:u16[][])  [unwired: 6 in, 2 out]
                            n220 = property on="Captured Image" class="IntGraph (strict)"("Value"=w395) -> ()  [unwired: 2 in, 2 out]
                          }
                          frame #2 {
                            # "ALWAYS free memory\nafter calling Async Grab\n(calls malloc)"
                            n221 = property on="pBuf address" class="DigNum (strict)"() -> ("Value"=w401:u32)  [unwired: 2 in, 2 out]
                            n222 = property on="pFrame address" class="DigNum (strict)"() -> ("Value"=w402:u32)  [unwired: 2 in, 2 out]
                            n223 = dll-call lib="C:/Users/appli/Documents/Aline/octo-labview/QImaging/Release/QImaging.dll" fn="RemFrame"(path in=w400, "pFrame"=w402, "pBuf"=w401) -> ()  [unwired: 5 in, 2 out]
                          }
                          frame #3 {
                            # "Save data"
                            n224 = property on="Save Data" class="Bool (strict)"() -> ("Value"=w404:bool)  [unwired: 2 in, 2 out]
                            n225 = case shown="True" w404 {
                              tunnel: w403 -> [_ w408]
                              frame False {
                              }
                              frame True {
                                n226 = property on="Indice" class="DigNum (strict)"() -> ("Value"=w410:u32)  [unwired: 2 in, 2 out]
                                n227 = property on="Overwrite?" class="Bool (strict)"() -> ("Value"=w411:bool)  [unwired: 2 in, 2 out]
                                n228 = property on="Nom du fichier" class="Str"() -> ("Value"=w409:string)  [unwired: 2 in, 2 out]
                                n229 = property on="Racine chemin de sauvegarde" class="Path"() -> ("Value"=w405:path)  [unwired: 2 in, 2 out]
                                n230 = call "CheckMonthDateFolder.vi"("Overwrite?"=w411, "Index"=w410, "File Name"=w409, "Folder Path Control"=w405) -> ("Warning"=w413:bool, "Message"=w412:string, "File Path"=w406:path)  [unwired: 5 in]
                                n231 = property on="Message" class="Str"("Value"=w412) -> ()  [unwired: 2 in, 2 out]
                                n232 = property on="Warning" class="Bool (strict)"("Value"=w413) -> ()  [unwired: 2 in, 2 out]
                                n233 = Not A Number/Path/Refnum?(number/path/refnum=w406) -> (NaN/Path/Refnum?=w407:bool)
                                n234 = case shown="False" w407 {
                                tunnel: w408 -> [w415 _]
                                tunnel: w406 -> [w416 _]
                                tunnel: w405 -> [w414 _]
                                frame False {
                                n235 = stacked-sequence {
                                seq-local: [w417 _ _] -> [_ w428 w432]
                                tunnel: w416 -> [w418 _ _]
                                tunnel: w415 -> [w419 _ _]
                                tunnel: w414 -> [_ _ w437]
                                frame #0 {
                                w423 = T4 7 items=["Grayscale (U8)", "Grayscale (I16)", "Grayscale (SGL)", "Complex (CSG)", "RGB (U32)", "HSL (U32)", "RGB (U64)", "Grayscale (U16)"] ("Image Type")
                                n236 = call "IMAQ Create"("Image Name"="", "Image Type"=w423) -> ("New Image"=w426:T5, "error out"=w420:errorcluster)  [unwired: 3 in]
                                n237 = call "IMAQ ArrayToImage"("Image Pixels (U16)"=w419, "error in (no error)"=w420, "Image"=w426) -> ("error out"=w421:errorcluster, "Image Out"=w427:T5)  [unwired: 7 in]
                                n238 = call-poly "IMAQ Write File 2"("error in (no error)"=w421, "File Path"=w418, "Image"=w427) -> ("error out"=w422:errorcluster, "Image Out (duplicate)"=w425:T5)  [unwired: 7 in]
                                n239 = call "IMAQ Dispose"("Image"=w425, "error in (no error)"=w422) -> ("error out"=w417:errorcluster)  [unwired: 4 in]
                                }
                                frame #1 {
                                n240 = case shown="No Error" w428 {
                                frame No Error {
                                # "incrémente si mode \nautomatique et écriture \nok"
                                n241 = property on="Mode de Sauvegarde" class="Ring (strict)"() -> ("Value"=w430:u16)  [unwired: 2 in, 2 out]
                                n242 = property on="Indice" class="DigNum (strict)"() -> ("Value"=w431:u32)  [unwired: 2 in, 2 out]
                                n243 = Add(x=w431, y=w430) -> (x+y=w429:u32)
                                n244 = property on="Indice" class="DigNum (strict)"("Value"=w429) -> ()  [unwired: 2 in, 2 out]
                                }
                                frame Error {
                                }
                                }
                                }
                                frame #2 {
                                # "Ecrit temps d'expo \ndans fichier de \ndonnées"
                                n245 = property on="Exposure Time" class="DigNum (strict)"() -> ("Value"=w433:u32)  [unwired: 2 in, 2 out]
                                n246 = property on="Nom du fichier" class="Str"() -> ("Value"=w438:string)  [unwired: 2 in, 2 out]
                                n247 = property on="Indice" class="DigNum (strict)"() -> ("Value"=w434:u32)  [unwired: 2 in, 2 out]
                                n248 = Build Path(base path=w437, name or relative path="Exposure.dat") -> (appended path=w435:path)
                                n249 = case shown="No Error" w432 {
                                tunnel: w438 -> [w445 _]
                                tunnel: w435 -> [w444 _]
                                tunnel: w434 -> [w443 _]
                                tunnel: w433 -> [w442 _]
                                frame No Error {
                                n250 = call "SavePictureData.vi"("File Path"=w444, "Exposure"=w442, "Index"=w443, "Name"=w445) -> ("error out"=w441:errorcluster)  [unwired: 7 in]
                                n251 = Unbundle By Name(w441) -> ("code"=w440:i32, "source"=w439:string)  [unwired: 1 out]
                                n252 = call <vilib>:"General Error Handler.vi"("[error code] (0)"=w440, "[error source] (\" \")"=w439) -> ()  [unwired: 9 in, 5 out]
                                }
                                frame Error {
                                }
                                }
                                }
                                }
                                }
                                frame True {
                                }
                                }
                              }
                            }
                          }
                          frame #4 {
                            # "Stats"
                            n253 = call "2DStatistics.vi"("data"=w448) -> ("Average"=w446:dbl, "StDev"=w447:dbl)  [unwired: 9 in]
                            n254 = property on="Average" class="DigNum (strict)"("Value"=w446) -> ()  [unwired: 2 in, 2 out]
                            n255 = property on="Std Dev" class="DigNum (strict)"("Value"=w447) -> ()  [unwired: 2 in, 2 out]
                            n256 = Array Max & Min(array=w448) -> (max value=w449:u16)  [unwired: 3 out]
                            n257 = property on="Max Val" class="DigNum (strict)"("Value"=w449) -> ()  [unwired: 2 in, 2 out]
                            n258 = Greater Or Equal?(x=w449, y=u16 16000) -> (x >= y?=w450:bool)
                            n259 = property on="Saturating?" class="Bool (strict)"("Value"=w450) -> ()  [unwired: 2 in, 2 out]
                          }
                        }
                      }
                      event "Abort Multi Grab": Value Change {
                        w458 = TRUE
                        n260 = event-data() -> ()  [unwired: 1 in, 6 out]
                        n261 = property on="Camera Handle" class="DigNum (strict)"() -> ("Value"=w464:u32)  [unwired: 2 in, 2 out]
                        n262 = call "QI_AbortFrame.vi"("path to dll"=w452, "error in (no error)"=w455, "Camera Handle"=w464) -> ("error out"=w454:errorcluster, "Camera Handle"=w460:u32)  [unwired: 7 in]
                        n263 = property on="pFrame address" class="DigNum (strict)"() -> ("Value"=w457:u32)  [unwired: 2 in, 2 out]
                        n264 = property on="pBuf address" class="DigNum (strict)"() -> ("Value"=w456:u32)  [unwired: 2 in, 2 out]
                        n265 = dll-call lib="C:/Users/appli/Documents/Aline/octo-labview/QImaging/Release/QImaging.dll" fn="RemFrame"(path in=w452, error in=w454, "pFrame"=w457, "pBuf"=w456) -> (error out=w453:errorcluster)  [unwired: 4 in, 1 out]
                        n266 = call "QI_ToggleStreaming.vi"("path to dll"=w452, "error in (no error)"=w453, "Enable?"=enum16{"Disable", "Enable"}."Disable", "Camera Handle"=w460) -> ("error out"=w459:errorcluster, "enable"=w461:u32)  [unwired: 4 in, 2 out]
                        n267 = Not Equal To 0?(x=w461) -> (x != 0?=w462:bool)
                        n268 = property on="Waiting for Trigger" class="Bool (strict)"("Value"=w462) -> ()  [unwired: 2 in, 2 out]
                      }
                    }
                  }
                }
                n269 = Unregister For Events(event registration refnum=w361) -> ()  [unwired: 1 in, 1 out]
              }
              frame #3 {
                n270 = property on="Abort Multi Grab" class="Bool"("DisabledEnum"=T2."Disabled and Grayed Out" ("Disabled")) -> ()  [unwired: 2 in, 2 out]
              }
            }
          }
          event "Stop": Value Change {
            n271 = event-data() -> ()  [unwired: 1 in, 6 out]
            n272 = flat-sequence {
              tunnel: w469 -> [w471]
              tunnel: w466 -> [w470]
              tunnel: [w473] -> w468
              tunnel: w466 -> [w472]
              frame #0 {
                n273 = call "QI_CloseCam.vi"("Camera Handle"=w471, "path to dll"=w470) -> ()  [unwired: 1 in, 3 out]
              }
              frame #1 {
                n274 = call "QI_CloseLib.vi"("path to dll"=w472) -> ("error out"=w473:errorcluster)  [unwired: 1 in, 1 out]
              }
            }
          }
          event "Exposure Time": Value Change {
            n275 = event-data() -> ()  [unwired: 1 in, 6 out]
            n276 = property on="Exposure Time" class="DigNum (strict)"() -> ("Value"=w478:u32)  [unwired: 2 in, 2 out]
            n277 = call "QI_ConfigCam.vi"("Camera Handle"=w477, "Parameter"=Parameter."Exposure", "paramVal"=w478, "error in (no error)"=w476, "path to dll"=w474) -> ("error out"=w475:errorcluster)  [unwired: 12 in, 2 out]
          }
          event Value Change {
            n278 = event-data() -> ()  [unwired: 1 in, 6 out]
            n279 = local read "Readout Speed"() -> (w483:T1)
            n280 = call "QI_ConfigCam.vi"("Camera Handle"=w485, "Parameter"=Parameter."Readout speed", "Readout Speed"=w483, "error in (no error)"=w482, "path to dll"=w480) -> ("error out"=w481:errorcluster)  [unwired: 12 in, 2 out]
          }
          event "Binning": Value Change {
            w492 = Parameter."Binning" ("Parameter")
            n281 = event-data() -> ("NewVal"=w491:u32)  [unwired: 1 in, 5 out]
            n282 = property on="CCD Height" class="DigNum (strict)"() -> ("Value"=w489:u32)  [unwired: 2 in, 2 out]
            n283 = property on="CCD Width" class="DigNum (strict)"() -> ("Value"=w490:u32)  [unwired: 2 in, 2 out]
            n284 = call "QI_ConfigCam.vi"("Camera Handle"=w502, "Parameter"=w492, "paramVal"=w491, "error in (no error)"=w501, "path to dll"=w486, "CCD Width"=w490, "CCD Height"=w489) -> ("Camera Handle"=w493:u32, "error out"=w494:errorcluster)  [unwired: 10 in, 1 out]
            n285 = call "QI_ConfigCam.vi"("Camera Handle"=w493, "Parameter"=w492, "paramVal"=w491, "error in (no error)"=w494, "path to dll"=w486, "CCD Width"=w490, "CCD Height"=w489) -> ("Camera Handle"=w488:u32, "error out"=w487:errorcluster)  [unwired: 10 in, 1 out]
            n286 = for {
              N: 6 -> [_]
              shift-right: [w509] -> w500
              shift-left: w487 -> [w513]
              tunnel: [w508] -> _
              tunnel: [w507] -> w499 mode=indexing
              tunnel: [w506] -> _ mode=indexing
              tunnel: w488 -> [w505]
              tunnel: w486 -> [w504]
              i -> [w512]
              n287 = Add(x=u32 8, y=w512) -> (x+y=w510:u32)
              n288 = call "QI_GetCamInfo.vi"("path to dll"=w504, "error in (no error)"=w513, "paramKey"=w510, "Camera Handle"=w505) -> ("error out"=w509:errorcluster, "CamInfo err"=w506:i32, "paramVal"=w507:u32, "Camera Handle"=w508:u32)  [unwired: 4 in]
            }
            n289 = Index Array(array=w499, index #1=0 ("index"), index #2=1 ("index")) -> (element #1=w495:u32, element #2=w496:u32)
            n290 = property on="ParamVal" class="Arr (strict)"("Value"=w499) -> ()  [unwired: 2 in, 2 out]
            n291 = property on="ROI Height" class="DigNum (strict)"("Value"=w496) -> ()  [unwired: 2 in, 2 out]
            n292 = property on="ROI Width" class="DigNum (strict)"("Value"=w495) -> ()  [unwired: 2 in, 2 out]
          }
          event "Trig": Value Change {
            n293 = event-data() -> ("NewVal"=w519:bool)  [unwired: 1 in, 5 out]
            n294 = Boolean To (0,1)(Boolean=w519) -> (0, 1=w520:i16)
            n295 = To Unsigned Long Integer(number=w520) -> (unsigned 32bit integer=w517:u32)
            n296 = call "QI_ConfigCam.vi"("Camera Handle"=w516, "Parameter"=Parameter."Trigger Type", "paramVal"=w517, "error in (no error)"=w518, "path to dll"=w514) -> ("error out"=w515:errorcluster)  [unwired: 12 in, 2 out]
          }
        }
        n297 = Compound Arithmetic op=OR(w138, w137) -> (w139:bool)
      }
    }
  }
  n298 = property on="Camera Handle" class="DigNum (strict)"() -> ("Value"=w2:u32)  [unwired: 2 in, 2 out]
  n299 = call "QI_ToggleStreaming.vi"("Enable?"=enum16{"Disable", "Enable"}."Disable", "Camera Handle"=w2) -> ("enable"=w4:u32)  [unwired: 6 in, 3 out]
  n300 = Not Equal To 0?(x=w4) -> (x != 0?=w3:bool)
  n301 = property on="Waiting for Trigger" class="Bool (strict)"("Value"=w3) -> ()  [unwired: 2 in, 2 out]
  n302 = flat-sequence {
    tunnel: w5 -> [w523]
    frame #0 {
      n303 = property on="Stop" class="Bool (strict)"("Value"=FALSE ("Stop")) -> ()  [unwired: 2 in, 2 out]
      n304 = property on="error out" class="Clust (strict)"("Value"=w523) -> ()  [unwired: 2 in, 2 out]
    }
  }
